vi "Create_Broadcast_News.vi"() -> (1 "News":string, 3 "广播？":bool)   [LabVIEW 2015]
uses:
  Database_util/Ctl/database_Method.ctl
  Database_util/Ctl/DNS.ctl
  Global/SeverGlobal.vi
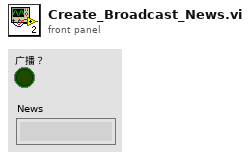
[diagram p1: front panel]
types:
  T1 = typedef "database_Method.ctl" = enum16{"初始化", "查询", "关闭"}
  T2 = typedef "DNS.ctl" = string
  T3 = cluster{"TCP Ref":refnum<k5>, "IP":string, "userName":string, "A":u16, "COM":u16, "time":u32}[]
  T4 = cluster{"TCP Ref":refnum<k5>, "Broadcast":refnum<k5>, "TF Ref":refnum<k5>, "IP":string, "port":u16, "userName":string, "passWord":string, "authority":string}[]
  T5 = cluster{"TCP Ref":refnum<k5>, "IP":string, "userName":string, "IN":u16, "OUT":u16, "time":u32}[]
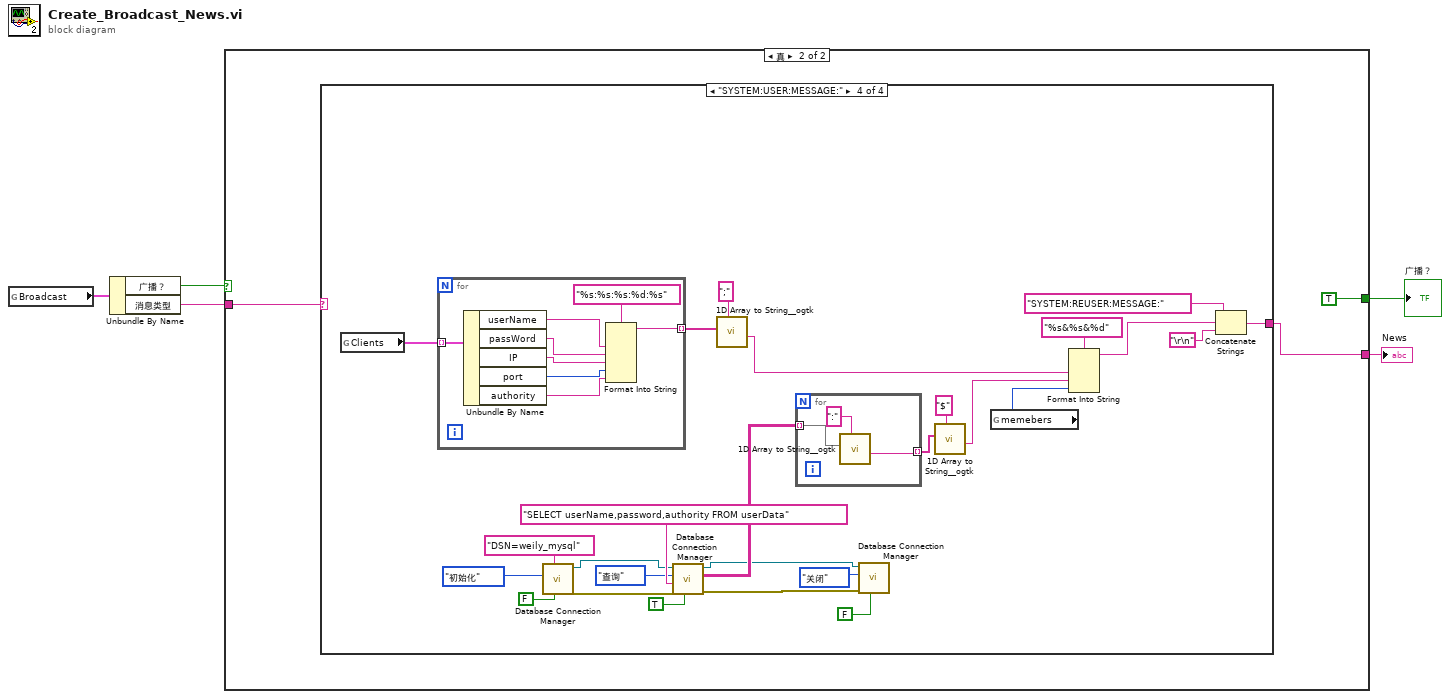
[diagram p0: block diagram]
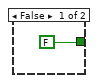
[diagram p2: hidden frame]
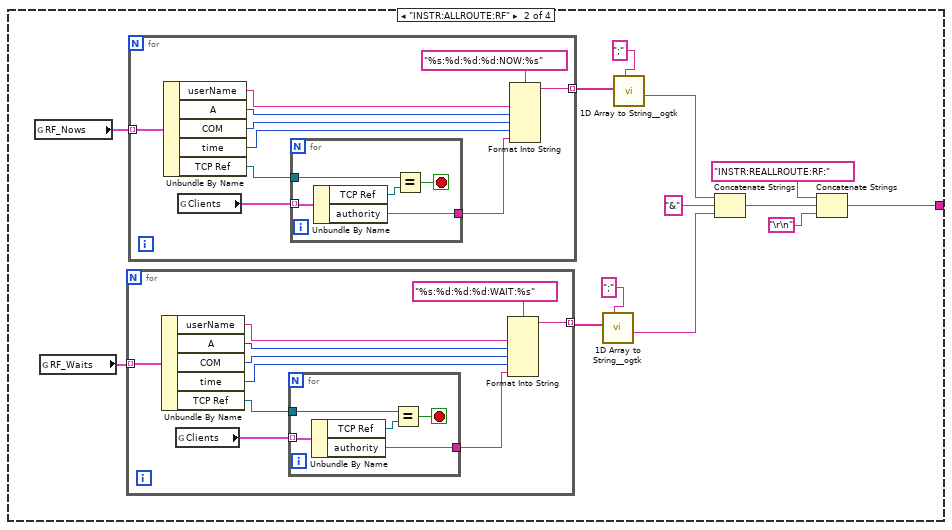
[diagram p4: hidden frame]
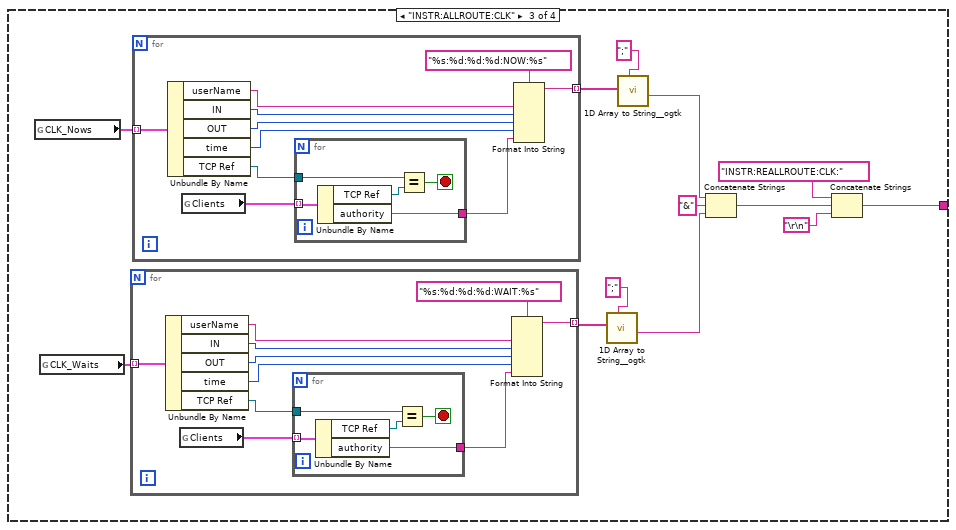
[diagram p5: hidden frame]
diagram:
  n1 = global read "SeverGlobal.vi" "Broadcast"() -> (w5:cluster{"消息类型":string, "广播？":bool})
  n2 = Unbundle By Name(w5) -> ("广播？"=w4:bool, "消息类型"=w2:string)
  n3 = case shown="真" w4 {
    tunnel: [FALSE ("广播？") TRUE ("广播？")] -> w3
    tunnel: w2 -> [_ w8]
    tunnel: [_ w7] -> w1
    frame False {
    }
    frame True {
      n4 = case shown="\"SYSTEM:USER:MESSAGE:\"" w8 {
        tunnel: [_ w10 w53 w105] -> w7
        frame Default {
        }
        frame "INSTR:ALLROUTE:RF" {
          n5 = global read "SeverGlobal.vi" "RF_Nows"() -> (w22:T3)
          n6 = global read "SeverGlobal.vi" "RF_Waits"() -> (w19:T3)
          n7 = for {
            tunnel: w19 -> [w32] mode=indexing
            tunnel: [w23] -> w17 mode=indexing
            n8 = Unbundle By Name(w32) -> ("userName"=w28:string, "A"=w27:u16, "COM"=w26:u16, "time"=w25:u32, "TCP Ref"=w30:refnum<k5>)
            n9 = global read "SeverGlobal.vi" "Clients"() -> (w31:T4)
            n10 = for {
              tunnel: w31 -> [w37] mode=indexing
              tunnel: w30 -> [w36]
              tunnel: [w33] -> w24
              stop <- w34 stop-if-true
              n11 = Unbundle By Name(w37) -> ("TCP Ref"=w35:refnum<k5>, "authority"=w33:string)
              n12 = Equal?(x=w36, y=w35) -> (x = y?=w34:bool)
            }
            n13 = Format Into String(format string="%s:%d:%d:%d:WAIT:%s", w28, w27, w26, w25, w24) -> (resulting string=w23:string)  [unwired: 2 in, 1 out]
          }
          n14 = for {
            tunnel: w22 -> [w47] mode=indexing
            tunnel: [w38] -> w20 mode=indexing
            n15 = Unbundle By Name(w47) -> ("userName"=w43:string, "A"=w42:u16, "COM"=w41:u16, "time"=w40:u32, "TCP Ref"=w45:refnum<k5>)
            n16 = global read "SeverGlobal.vi" "Clients"() -> (w46:T4)
            n17 = for {
              tunnel: w46 -> [w52] mode=indexing
              tunnel: w45 -> [w51]
              tunnel: [w48] -> w39
              stop <- w49 stop-if-true
              n18 = Unbundle By Name(w52) -> ("TCP Ref"=w50:refnum<k5>, "authority"=w48:string)
              n19 = Equal?(x=w51, y=w50) -> (x = y?=w49:bool)
            }
            n20 = Format Into String(format string="%s:%d:%d:%d:NOW:%s", w43, w42, w41, w40, w39) -> (resulting string=w38:string)  [unwired: 2 in, 1 out]
          }
          n21 = call <userlib>:"1D Array to String__ogtk.vi"("delimiter (Tab)"=";", "Array of Strings"=w17) -> ("delimited string"=w14:string)  [unwired: 9 in]
          n22 = call <userlib>:"1D Array to String__ogtk.vi"("delimiter (Tab)"=";", "Array of Strings"=w20) -> ("delimited string"=w15:string)  [unwired: 9 in]
          n23 = Concatenate Strings(w15, "&" ("string"), w14) -> (w11:string)
          n24 = Concatenate Strings("INSTR:REALLROUTE:RF:" ("regular expression"), w11, "\r\n") -> (w10:string)
        }
        frame "INSTR:ALLROUTE:CLK" {
          n25 = global read "SeverGlobal.vi" "CLK_Nows"() -> (w65:T5)
          n26 = global read "SeverGlobal.vi" "CLK_Waits"() -> (w62:T5)
          n27 = for {
            tunnel: w62 -> [w75] mode=indexing
            tunnel: [w66] -> w60 mode=indexing
            n28 = Unbundle By Name(w75) -> ("userName"=w71:string, "IN"=w70:u16, "OUT"=w69:u16, "time"=w68:u32, "TCP Ref"=w73:refnum<k5>)
            n29 = global read "SeverGlobal.vi" "Clients"() -> (w74:T4)
            n30 = for {
              tunnel: w74 -> [w80] mode=indexing
              tunnel: w73 -> [w79]
              tunnel: [w76] -> w67
              stop <- w77 stop-if-true
              n31 = Unbundle By Name(w80) -> ("TCP Ref"=w78:refnum<k5>, "authority"=w76:string)
              n32 = Equal?(x=w79, y=w78) -> (x = y?=w77:bool)
            }
            n33 = Format Into String(format string="%s:%d:%d:%d:WAIT:%s", w71, w70, w69, w68, w67) -> (resulting string=w66:string)  [unwired: 2 in, 1 out]
          }
          n34 = for {
            tunnel: w65 -> [w90] mode=indexing
            tunnel: [w81] -> w63 mode=indexing
            n35 = Unbundle By Name(w90) -> ("userName"=w86:string, "IN"=w85:u16, "OUT"=w84:u16, "time"=w83:u32, "TCP Ref"=w88:refnum<k5>)
            n36 = global read "SeverGlobal.vi" "Clients"() -> (w89:T4)
            n37 = for {
              tunnel: w89 -> [w95] mode=indexing
              tunnel: w88 -> [w94]
              tunnel: [w91] -> w82
              stop <- w92 stop-if-true
              n38 = Unbundle By Name(w95) -> ("TCP Ref"=w93:refnum<k5>, "authority"=w91:string)
              n39 = Equal?(x=w94, y=w93) -> (x = y?=w92:bool)
            }
            n40 = Format Into String(format string="%s:%d:%d:%d:NOW:%s", w86, w85, w84, w83, w82) -> (resulting string=w81:string)  [unwired: 2 in, 1 out]
          }
          n41 = call <userlib>:"1D Array to String__ogtk.vi"("delimiter (Tab)"=";", "Array of Strings"=w60) -> ("delimited string"=w57:string)  [unwired: 9 in]
          n42 = call <userlib>:"1D Array to String__ogtk.vi"("delimiter (Tab)"=";", "Array of Strings"=w63) -> ("delimited string"=w58:string)  [unwired: 9 in]
          n43 = Concatenate Strings(w58, "&" ("string"), w57) -> (w54:string)
          n44 = Concatenate Strings("INSTR:REALLROUTE:CLK:" ("regular expression"), w54, "\r\n") -> (w53:string)
        }
        frame "SYSTEM:USER:MESSAGE:" {
          n45 = global read "SeverGlobal.vi" "Clients"() -> (w106:T4)
          n46 = for {
            tunnel: w106 -> [w132] mode=indexing
            tunnel: [w125] -> w115 mode=indexing
            n47 = Unbundle By Name(w132) -> ("userName"=w130:string, "passWord"=w129:string, "IP"=w128:string, "port"=w127:u16, "authority"=w126:string)
            n48 = Format Into String(format string="%s:%s:%s:%d:%s", w130, w129, w128, w127, w126) -> (resulting string=w125:string)  [unwired: 2 in, 1 out]
          }
          n49 = call "Database Connection Manager.vi"("Return Data (T)"=FALSE, "ConnectionString"=T2 "DSN=weily_mysql", "Method"=database_Method."初始化") -> ("error out"=w101:errorcluster, "ADODB._Connection Out"=w102:refnum<k7>)  [unwired: 5 in, 2 out]
          n50 = call "Database Connection Manager.vi"("Return Data (T)"=TRUE, "error in (no error)"=w101, "Command Text"="SELECT userName,password,authority FROM userData" ("SQL"), "Method"=database_Method."查询", "ADODB._Connection In"=w102) -> ("error out"=w100:errorcluster, "Data"=w118:string[][], "ADODB._Connection Out"=w98:refnum<k7>)  [unwired: 3 in, 1 out]
          n51 = call <userlib>:"1D Array to String__ogtk.vi"("delimiter (Tab)"=";", "Array of Strings"=w115) -> ("delimited string"=w117:string)  [unwired: 9 in]
          n52 = for {
            tunnel: w118 -> [w124] mode=indexing
            tunnel: [w122] -> w119 mode=indexing
            n53 = call <userlib>:"1D Array to String__ogtk.vi"("delimiter (Tab)"=":", "Array of Strings"=w124) -> ("delimited string"=w122:string)  [unwired: 9 in]
          }
          n54 = call "Database Connection Manager.vi"("Return Data (T)"=FALSE, "error in (no error)"=w100, "Method"=database_Method."关闭", "ADODB._Connection In"=w98) -> ()  [unwired: 4 in, 4 out]
          n55 = call <userlib>:"1D Array to String__ogtk.vi"("delimiter (Tab)"="$", "Array of Strings"=w119) -> ("delimited string"=w121:string)  [unwired: 9 in]
          n56 = global read "SeverGlobal.vi" "memebers"() -> (w112:i32)
          n57 = Format Into String(format string="%s&%s&%d", w117, w121, w112) -> (resulting string=w114:string)  [unwired: 2 in, 1 out]
          n58 = Concatenate Strings("SYSTEM:REUSER:MESSAGE:", w114, "\r\n") -> (w105:string)
        }
      }
    }
  }
  "广播？" <- w3
  "News" <- w1
